vi "nelder_calculate_area.vi"() -> ()   [LabVIEW 2018]
panel:
  out "transposed array":sgl[][](array[numeric])
  in  "next simplex":sgl[][](array[numeric])
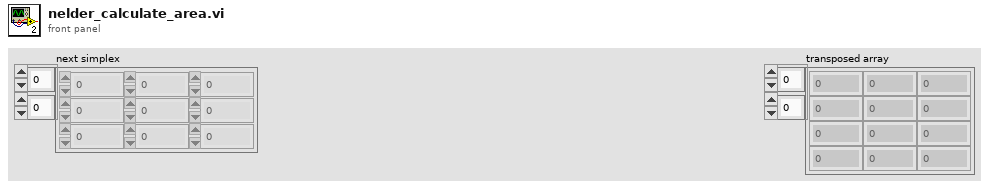
[diagram p1: front panel]
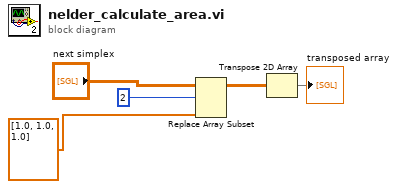
[diagram p0: block diagram]
diagram:
  n1 = Replace Array Subset(array="next simplex", new element=sgl[] [1.0, 1.0, 1.0] ("new element/subarray"), index (row)=2) -> (w2:sgl[][])  [unwired: 1 in]
  n2 = Transpose 2D Array(2D array=w2) -> (transposed array=→"transposed array":sgl[][])
